vi "延时函数.vi"() -> ()   [LabVIEW 2017]
panel:
  out "t2":u32
  in  "t1":u32
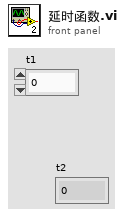
[diagram p1: front panel]
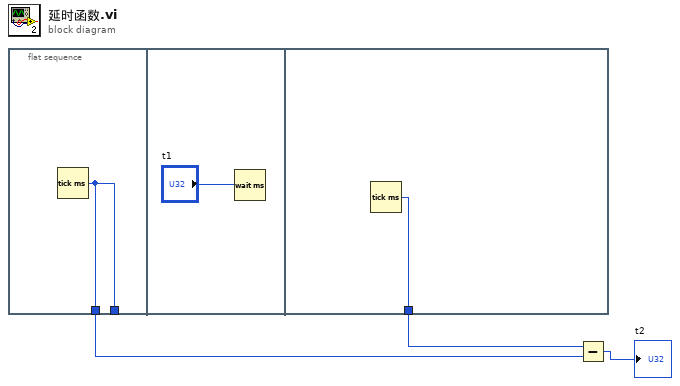
[diagram p0: block diagram]
diagram:
  n1 = flat-sequence {
    tunnel: [w4] -> _
    tunnel: [w4] -> w3
    tunnel: [w6] -> w2
    frame #0 {
      n2 = Tick Count (ms)() -> (millisecond timer value=w4:u32)
    }
    frame #1 {
      n3 = Wait (ms)(milliseconds to wait="t1") -> ()  [unwired: 1 out]
    }
    frame #2 {
      n4 = Tick Count (ms)() -> (millisecond timer value=w6:u32)
    }
  }
  n5 = Subtract(x=w2, y=w3) -> (x-y=→"t2":u32)
